vi "Get Device Information.vi"(11 "SOL MS in":refnum<class "PL SOL Instruments MS.lvclass">) -> (2 "info":T1, 3 "SOL MS out":refnum<class "PL SOL Instruments MS.lvclass">)   [LabVIEW 2015, in "PL SOL Instruments MS.lvclass"]
doc: "Returns device specification read from the configuration file."
uses:
  PL SOL Instruments MS.lvclass
  PL SOL Instruments MS.lvclass/PL SOL Instruments MS.ctl
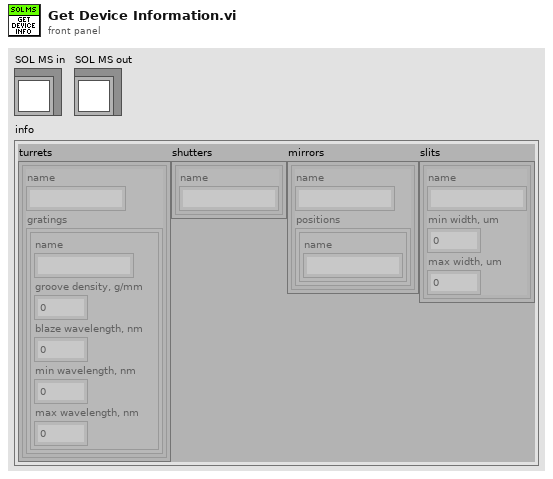
[diagram p1: front panel]
types:
  T1 = cluster{"turrets":cluster{"name":string, "gratings":cluster{"name":string, "groove density, g/mm":dbl, "blaze wavelength, nm":dbl, "min wavelength, nm":dbl, "max wavelength, nm":dbl}[]}[], "shutters":cluster{"name":string}[], "mirrors":cluster{"name":string, "positions":cluster{"name":string}[]}[], "slits":cluster{"name":string, "min width, um":dbl, "max width, um":dbl}[]}
  T2 = cluster{"name":string, "step timeout, ms":u32, "reset timeout, ms":u32, "gratings":cluster{"name":string, "step timeout, ms":u32, "reset timeout, ms":u32, "turret position":i32, "reset position":i32, "max position":i32, "backlash distance":i32, "step size, rad":dbl, "groove density, g/mm":dbl, "theta2, rad":dbl, "blaze wavelength, nm":dbl, "focal length, cm":dbl, "manual change":bool, "manual change position":i32}[], "current grating":cluster{"index":u8, "position":i32}}[]
  T3 = cluster{"name":string, "step timeout, ms":u32, "reset timeout, ms":u32, "positions":cluster{"name":string, "position":i32}[], "current position index":u8}[]
  T4 = cluster{"name":string, "step timeout, ms":u32, "reset position":i32, "max position":i32, "backlash distance":i32, "step size, um":dbl, "current position":i32}[]
  T5 = cluster{"name":string, "gratings":cluster{"name":string, "groove density, g/mm":dbl, "blaze wavelength, nm":dbl, "min wavelength, nm":dbl, "max wavelength, nm":dbl}[]}[]
  T6 = cluster{"name":string, "positions":cluster{"name":string}[]}[]
  T7 = cluster{"name":string, "min width, um":dbl, "max width, um":dbl}[]
  T8 = cluster{"name":string, "gratings":cluster{"name":string, "groove density, g/mm":dbl, "blaze wavelength, nm":dbl, "min wavelength, nm":dbl, "max wavelength, nm":dbl}[]}
  T9 = cluster{"name":string, "positions":cluster{"name":string}[]}
  T10 = cluster{"name":string, "min width, um":dbl, "max width, um":dbl}
  T11 = cluster{"name":string, "groove density, g/mm":dbl, "blaze wavelength, nm":dbl, "min wavelength, nm":dbl, "max wavelength, nm":dbl}[]
  T12 = cluster{"name":string, "groove density, g/mm":dbl, "blaze wavelength, nm":dbl, "min wavelength, nm":dbl, "max wavelength, nm":dbl}
  T13 = cluster{"name":string, "step timeout, ms":u32, "reset timeout, ms":u32, "turret position":i32, "reset position":i32, "max position":i32, "backlash distance":i32, "step size, rad":dbl, "groove density, g/mm":dbl, "theta2, rad":dbl, "blaze wavelength, nm":dbl, "focal length, cm":dbl, "manual change":bool, "manual change position":i32}[]
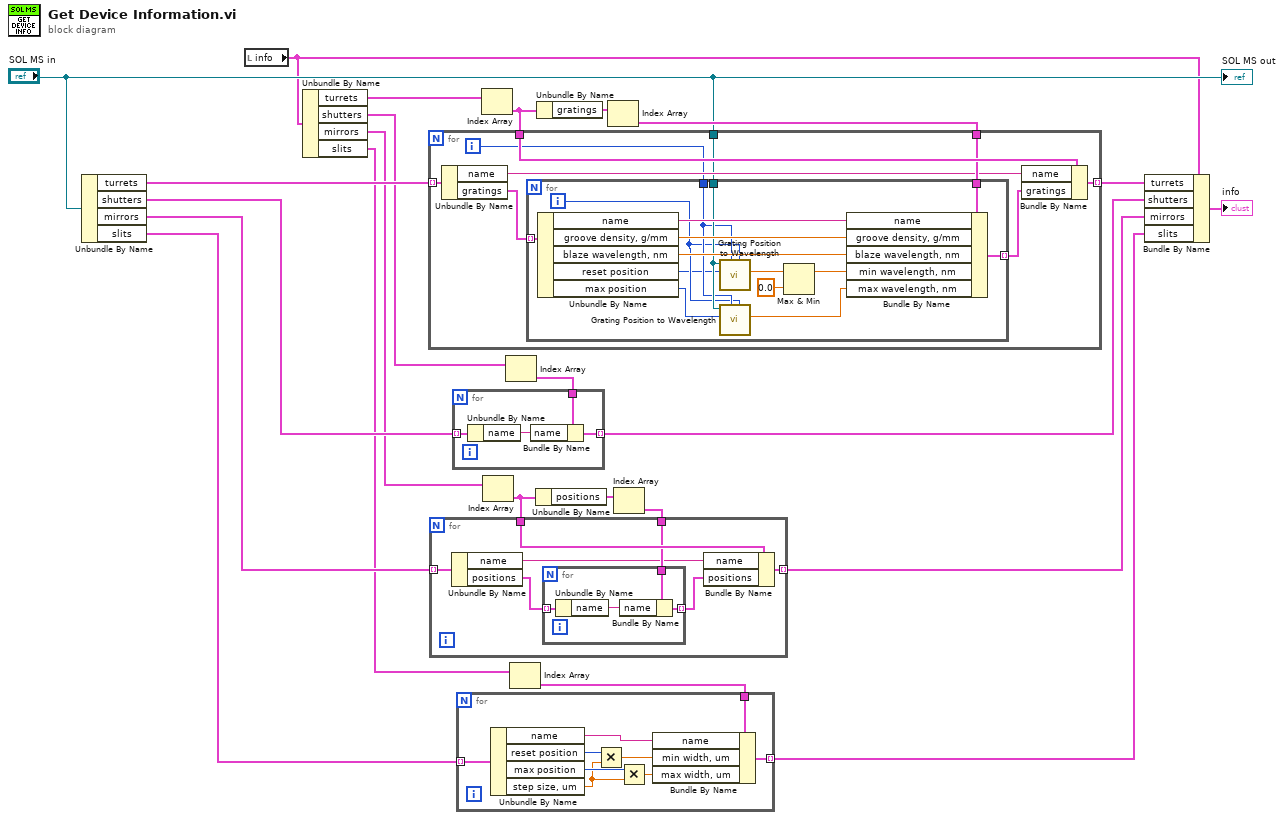
[diagram p0: block diagram]
diagram:
  n1 = Unbundle By Name("SOL MS in") -> ("turrets"=w20:T2, "shutters"=w14:cluster{"name":string, "is open":bool}[], "mirrors"=w16:T3, "slits"=w12:T4)
  n2 = local read "info"() -> (w2:T1)
  n3 = Unbundle By Name(w2) -> ("turrets"=w9:T5, "shutters"=w4:cluster{"name":string}[], "mirrors"=w8:T6, "slits"=w7:T7)
  n4 = Index Array(array=w9) -> (element=w22:T8)  [unwired: 1 in]
  n5 = Index Array(array=w8) -> (element=w18:T9)  [unwired: 1 in]
  n6 = Index Array(array=w4) -> (element=w15:cluster{"name":string})  [unwired: 1 in]
  n7 = for {
    tunnel: w15 -> [w27]
    tunnel: w14 -> [w26] mode=indexing
    tunnel: [w24] -> w10 mode=indexing
    n8 = Unbundle By Name(w26) -> ("name"=w25:string)
    n9 = Bundle By Name(cluster=w27, "name"=w25) -> (w24:cluster{"name":string})
  }
  n10 = Index Array(array=w7) -> (element=w13:T10)  [unwired: 1 in]
  n11 = for {
    tunnel: w13 -> [w36]
    tunnel: w12 -> [w35] mode=indexing
    tunnel: [w33] -> w6 mode=indexing
    n12 = Unbundle By Name(w35) -> ("name"=w34:string, "reset position"=w32:i32, "max position"=w30:i32, "step size, um"=w29:dbl)
    n13 = Multiply(x=w32, y=w29) -> (x*y=w31:dbl)
    n14 = Multiply(x=w30, y=w29) -> (x*y=w28:dbl)
    n15 = Bundle By Name(cluster=w36, "name"=w34, "min width, um"=w31, "max width, um"=w28) -> (w33:T10)
  }
  n16 = Unbundle By Name(w18) -> ("positions"=w17:cluster{"name":string}[])
  n17 = Unbundle By Name(w22) -> ("gratings"=w23:T11)
  n18 = Index Array(array=w23) -> (element=w21:T12)  [unwired: 1 in]
  n19 = for {
    tunnel: w22 -> [w45]
    tunnel: w21 -> [w44]
    tunnel: w20 -> [w43] mode=indexing
    tunnel: [w39] -> w11 mode=indexing
    tunnel: "SOL MS in" -> [w37]
    i -> [w38]
    n20 = Unbundle By Name(w43) -> ("name"=w42:string, "gratings"=w41:T13)
    n21 = for {
      tunnel: w44 -> [w60]
      tunnel: w41 -> [w59] mode=indexing
      tunnel: [w55] -> w40 mode=indexing
      tunnel: w38 -> [w49]
      tunnel: w37 -> [w52]
      i -> [w48]
      n22 = Unbundle By Name(w59) -> ("name"=w58:string, "groove density, g/mm"=w57:dbl, "blaze wavelength, nm"=w56:dbl, "reset position"=w47:i32, "max position"=w46:i32)
      n23 = call "Grating Position to Wavelength.vi"("grating index (0)"=w48, "turret index (0)"=w49, "grating position"=w47, "SOL MS in"=w52) -> ("wavelength, nm"=w50:dbl)  [unwired: 5 in, 2 out]
      n24 = call "Grating Position to Wavelength.vi"("grating index (0)"=w48, "turret index (0)"=w49, "grating position"=w46, "SOL MS in"=w52) -> ("wavelength, nm"=w51:dbl)  [unwired: 5 in, 2 out]
      n25 = Max & Min(x=w50, y=0.0) -> (max(x,y)=w53:dbl)  [unwired: 1 out]
      n26 = Bundle By Name(cluster=w60, "name"=w58, "groove density, g/mm"=w57, "blaze wavelength, nm"=w56, "min wavelength, nm"=w53, "max wavelength, nm"=w51) -> (w55:T12)
    }
    n27 = Bundle By Name(cluster=w45, "name"=w42, "gratings"=w40) -> (w39:T8)
  }
  n28 = Index Array(array=w17) -> (element=w19:cluster{"name":string})  [unwired: 1 in]
  n29 = for {
    tunnel: w18 -> [w67]
    tunnel: w19 -> [w66]
    tunnel: w16 -> [w65] mode=indexing
    tunnel: [w61] -> w5 mode=indexing
    n30 = Unbundle By Name(w65) -> ("name"=w64:string, "positions"=w63:cluster{"name":string, "position":i32}[])
    n31 = for {
      tunnel: w66 -> [w71]
      tunnel: w63 -> [w70] mode=indexing
      tunnel: [w68] -> w62 mode=indexing
      n32 = Unbundle By Name(w70) -> ("name"=w69:string)
      n33 = Bundle By Name(cluster=w71, "name"=w69) -> (w68:cluster{"name":string})
    }
    n34 = Bundle By Name(cluster=w67, "name"=w64, "positions"=w62) -> (w61:T9)
  }
  n35 = Bundle By Name(cluster=w2, "turrets"=w11, "shutters"=w10, "mirrors"=w5, "slits"=w6) -> (→"info":T1)
  "SOL MS out" <- "SOL MS in"
